vi "Write Layer index.vi"(8 "error in (no error)":errorcluster, 10 "Iteration/layer index":u16, 11 "Storage params in":refnum<class "CV-Storage.lvclass">) -> (0 "error out":errorcluster, 3 "Storage params out":refnum<class "CV-Storage.lvclass">)   [LabVIEW 2013, in "CameraVision.lvlib" / "CV-Storage.lvclass"]
uses:
  CV-Storage.lvclass
  CV-Storage.lvclass/CV-Storage.ctl
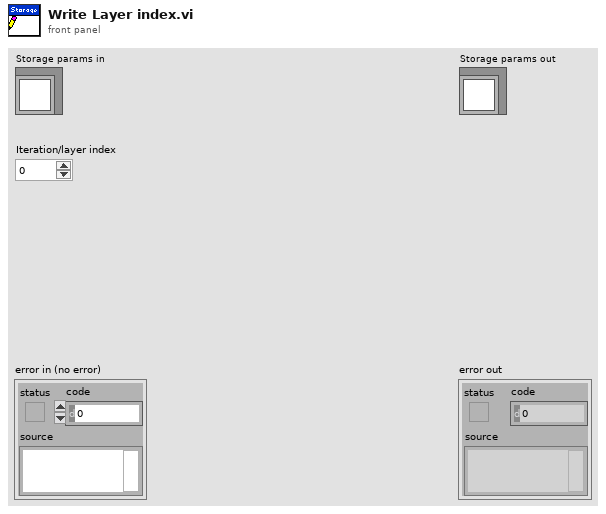
[diagram p1: front panel]
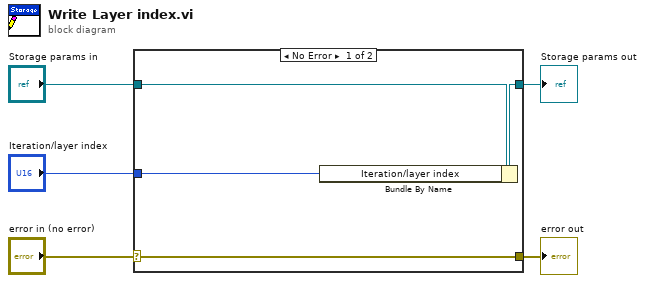
[diagram p0: block diagram]
diagram:
  n1 = case shown="No Error" "error in (no error)" {
    selector: "error in (no error)" -> [w9 w10]
    tunnel: [w9 w10] -> w4
    tunnel: [w7 w11] -> w2
    tunnel: "Storage params in" -> [w8 w11]
    tunnel: "Iteration/layer index" -> [w6 _]
    frame No Error {
      n2 = Bundle By Name(cluster=w8, "Iteration/layer index"=w6) -> (w7:refnum<class "CV-Storage.lvclass">)
    }
    frame Error {
    }
  }
  "error out" <- w4
  "Storage params out" <- w2
